vi "Main.vi"(11 "Module Admin":refnum<class "Delacor_lib_QMH_Module Admin.lvclass">) -> ()   [LabVIEW 2020, in "Logger.lvlib"]
doc: "This template is based off of the Queued Message Handler design pattern and the Queued Message Handler project template that ships with LabVIEW.\n\nThe main difference is that the queue is private to this module and communication between modules is performed via Broadcast and Request events.\n\nRequest events are wrapped in public API methods and are handled in the Event Handling Loop (EHL) of this VI. Any module can register for Broadcast events sent by this module. The EHL generates messages based on user interface actions.\n\nThe Message Handling Loop (MHL) processes messages generated by the EHL, or by other messages. The messages are string values, so new messages can be added easily to the Message Cases case structure in the MHL. Each message cluster can also provide an optional value for Message Data, which is a variant that can be converted to whatever message-specific data is required.\n_____\nBased on Delacor QMH Project Template 4.0.0.47.\n_____\nBased on DQMH Project Template 6.0.0.91."
uses:
  Logger.lvlib
  <vilib>/Delacor/Delacor QMH/Libraries/Module Admin_class/Delacor_lib_QMH_Module Admin.lvclass
  Module Data--cluster.ctl
  Stop Argument--cluster.ctl
  <vilib>/Delacor/Delacor QMH/Libraries/Message Queue_class/Delacor_lib_QMH_Message Queue.lvclass/Delacor_lib_QMH_Message Queue.ctl
  <vilib>/Delacor/Delacor QMH/Libraries/Module Admin_class/Delacor_lib_QMH_Module Admin.lvclass/Delacor_lib_QMH_Module Admin.ctl
  Initialize File Argument--cluster.ctl
  Initialize File (Reply Payload)--cluster.ctl
  Log Data Argument--cluster.ctl
  Stop Logging Argument--cluster.ctl
  Settings Editor/Update Application Settings (Reply Payload)--cluster.ctl
  Settings Editor/Settings--cluster.ctl
  Settings Editor/DAQmx Config--cluster.ctl
  Settings Editor/DAQmx Trigger Settings--cluster.ctl
  Settings Editor/DAQmx Timing--cluster.ctl
  Start Logging Argument--cluster.ctl
  <vilib>/Utility/miscctls.llb/LVPointTypeDef.ctl
  <vilib>/Delacor/Delacor QMH/Libraries/Message Queue_class/Delacor_lib_QMH_Enqueue Message (Single).vi
  <vilib>/Delacor/Delacor QMH/Libraries/Module Admin_class/Delacor_lib_QMH_Get External Launch.vi
  <vilib>/Utility/error.llb/Error Cluster From Error Code.vi
  <vilib>/ErrorRing/Error Ring.xnode
  <vilib>/Delacor/Delacor QMH/Libraries/Message Queue_class/Delacor_lib_QMH_Message Queue.lvclass
  Settings Editor/Settings Editor.lvlib
panel:
  out "Settings":T1
  out "error out":errorcluster
  # "This is a headless module. Show its panel to confirm that the Settings are updated correctly and other debugging tasks. Use the Settings Editor to change the settings for this module."
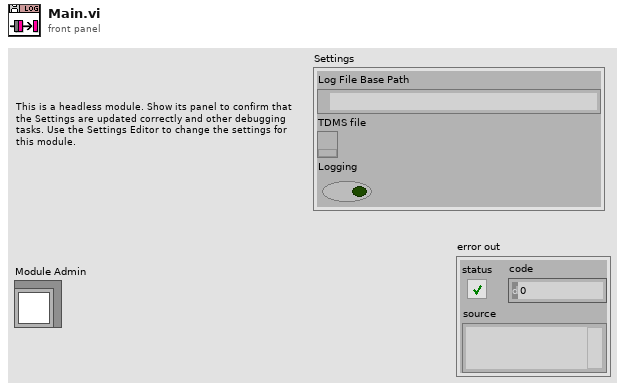
[diagram p1: front panel]
types:
  T1 = typedef "Logger.lvlib/Module Data--cluster.ctl" = cluster{"Log File Base Path":path, "TDMS file":refnum<k34>, "Logging":bool}
  T2 = typedef "Settings Editor.lvlib/Broadcast Events--cluster.ctl" = cluster{"Module Did Init":refnum<user-event>, "Status Updated":refnum<user-event>, "Error Reported":refnum<user-event>, "Module Did Stop":refnum<user-event>, "Update Module Execution Status":refnum<user-event>, "Application Settings Updated":refnum<user-event>}
  T3 = typedef "Logger.lvlib/Request Events--cluster.ctl" = cluster{"Stop Module":refnum<user-event>, "Show Panel":refnum<user-event>, "Hide Panel":refnum<user-event>, "Get Module Execution Status":refnum<user-event>, "Show Diagram":refnum<user-event>, "Stop Logging":refnum<user-event>, "Log Data":refnum<user-event>, "Initialize File":refnum<user-event>, "Start Logging":refnum<user-event>}
  T4 = enum32{"invalid lock state", "Not Locked", "Locked (No Password)", "Password-protected"}
  T5 = typedef "Logger.lvlib/Stop Argument--cluster.ctl" = cluster{"Origin":string, "Exit via Stop Module Req?":bool, "Wait for Module to stop?":bool}
  T6 = typedef "Logger.lvlib/Initialize File Argument--cluster.ctl" = cluster{"Wait Notifier":refnum<notifier>, "wait for reply":bool}
  T7 = typedef "Logger.lvlib/Log Data Argument--cluster.ctl" = cluster{"Waveforms":waveform(dbl)[]}
  T8 = typedef "Logger.lvlib/Stop Logging Argument--cluster.ctl" = cluster{"Boolean":bool}
  T9 = typedef "Settings Editor.lvlib/Update Application Settings (Reply Payload)--cluster.ctl" = cluster{"Settings":T10, "Update Settings_error":errorcluster}
  T10 = typedef "Settings Editor.lvlib/Settings--cluster.ctl" = cluster{"Calibration Array":cluster{"Slope":dbl, "Offset":dbl}[], "Hardware Config Cluster":T11, "Trigger Settings":T12, "Log File Base Path":path, "DAQmx Timing Settings":T13}
  T11 = typedef "Settings Editor.lvlib/DAQmx Config--cluster.ctl" = cluster{"Physical channels":tag, "Channel Name":string, "Unit":i32, "Min Voltage":dbl, "Max Voltage":dbl}[]
  T12 = typedef "Settings Editor.lvlib/DAQmx Trigger Settings--cluster.ctl" = cluster{"Trigger Type":enum32{"No Trigger", "Digital Start", "Digital Pause", "Digital Reference", "Analog Start", "Analog Pause", "Analog Reference", "Time Start"}, "Digital Start":cluster{"Source":tag, "Digital Start Trigger Edge":i32}, "Digital Pause":cluster{"Source":tag, "Digital Pause Trigger Pause When":i32}, "Digital Reference":cluster{"Source":tag, "Digital Start Trigger Edge":i32, "Digital Reference Pretrigger Samples":u32}, "Analog Start":cluster{"Source":string, "Analog Slope":i32, "Analog Start Trigger Hysteresis":dbl, "Analog Start Trigger Level":dbl}, "Analog Pause":cluster{"Source":string, "Analog Start Trigger Level":dbl, "Analog Pause Trigger Pause When":i32}, "Analog Reference":cluster{"Source":string, "Slope":i32, "Pretrigger Samples":u32, "Level":dbl}, "Time Start":cluster{"Select Time\nManually":bool, "When":timestamp}}
  T13 = typedef "Settings Editor.lvlib/DAQmx Timing--cluster.ctl" = cluster{"rate":dbl, "source":tag, "sample mode":i32, "samples per channel":i32}
  T14 = typedef "Logger.lvlib/Start Logging Argument--cluster.ctl" = cluster{"Boolean":bool}
  T15 = typedef "LVPointTypeDef.ctl" = cluster{"Horizontal":i16, "Vertical":i16}
  T16 = enum32{"Invalid", "Standard", "Closed", "Hidden", "Minimized", "Maximized"}
  T17 = typedef "Logger.lvlib/Initialize File (Reply Payload)--cluster.ctl" = cluster{"File Path":path, "Initialize File_error":errorcluster}
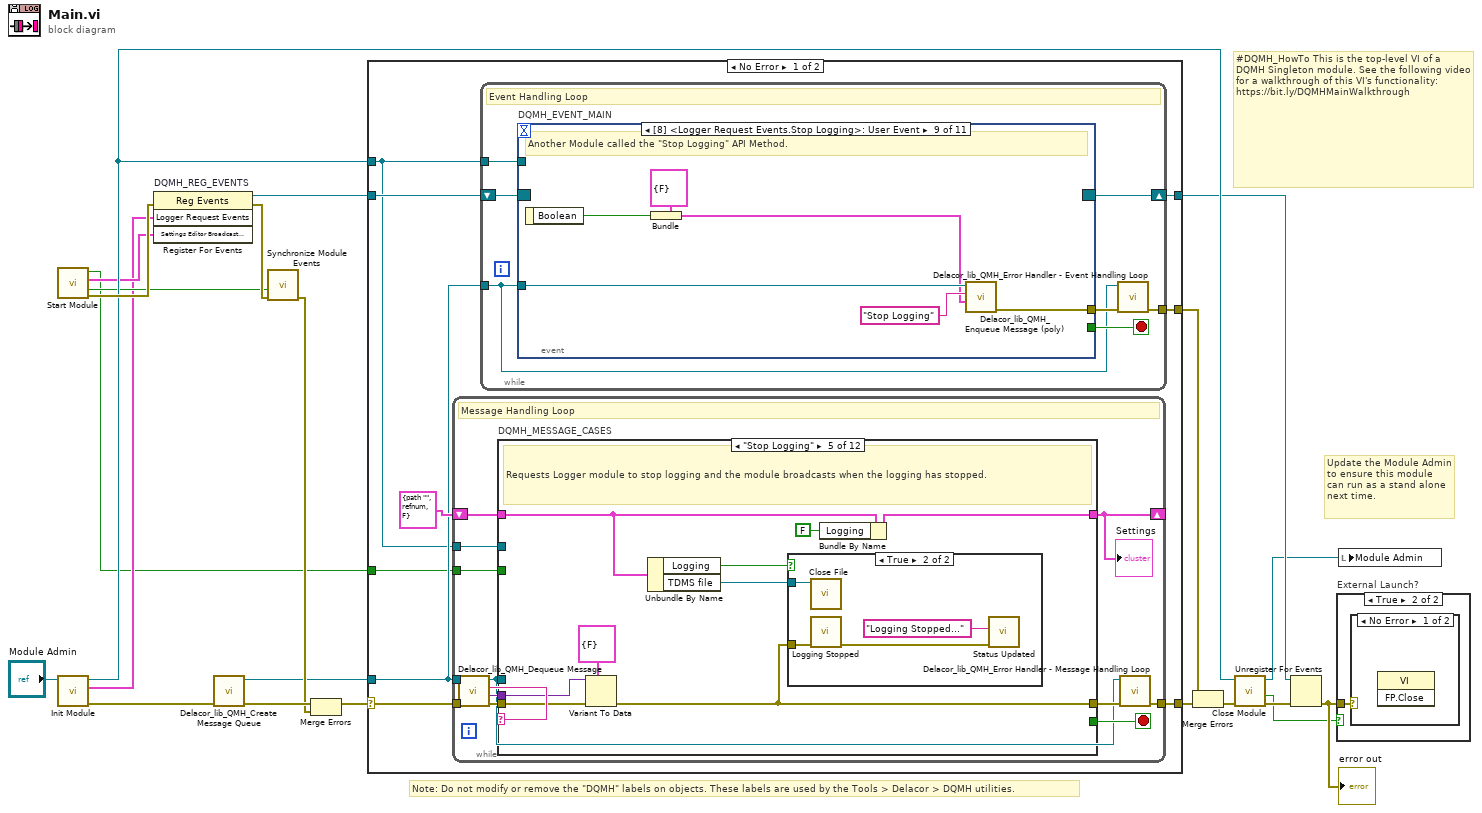
[diagram p0: block diagram]
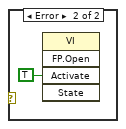
[diagram p3: hidden frame]
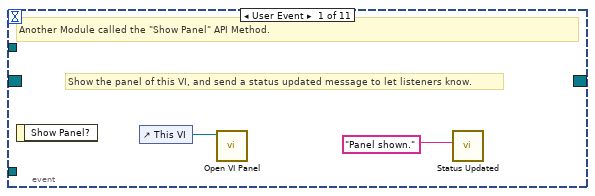
[diagram p4: hidden frame]
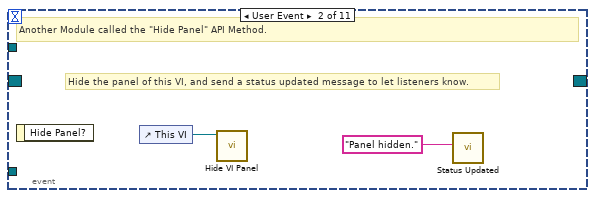
[diagram p5: hidden frame]
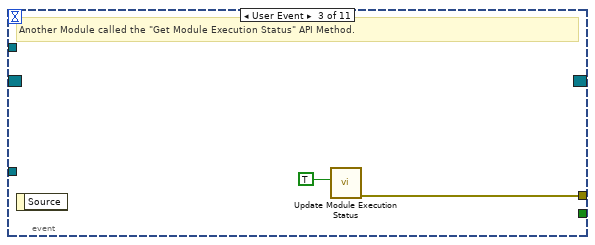
[diagram p6: hidden frame]
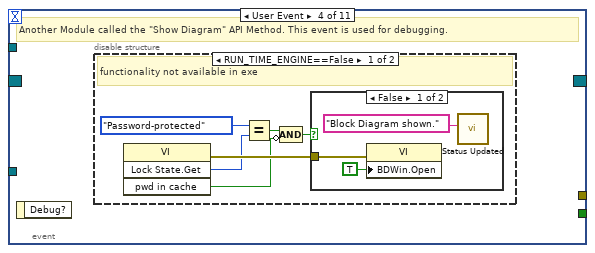
[diagram p7: hidden frame]
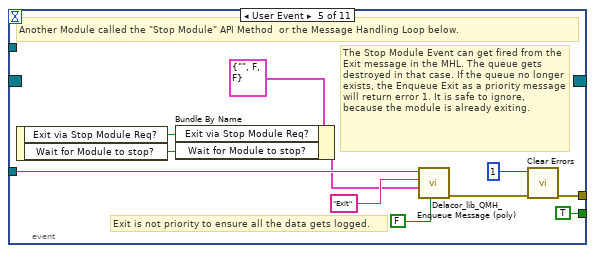
[diagram p10: hidden frame]
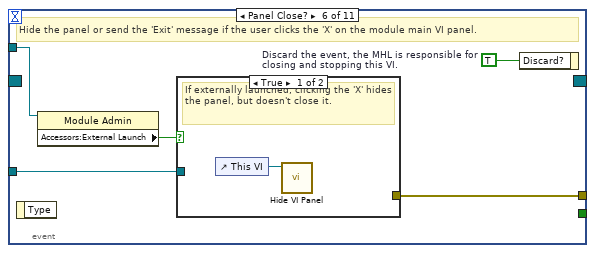
[diagram p11: hidden frame]
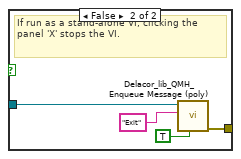
[diagram p12: hidden frame]
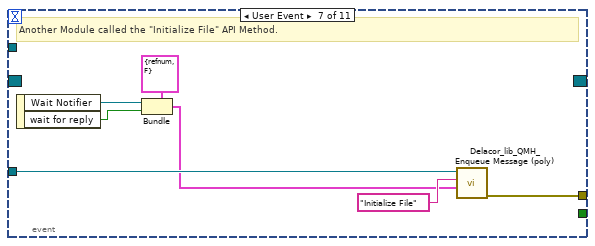
[diagram p13: hidden frame]
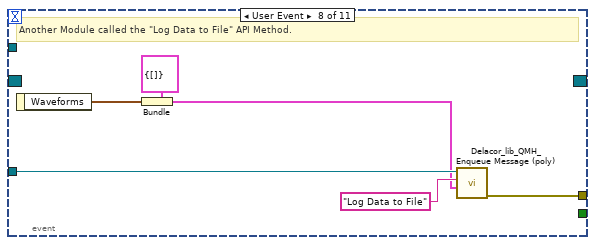
[diagram p14: hidden frame]
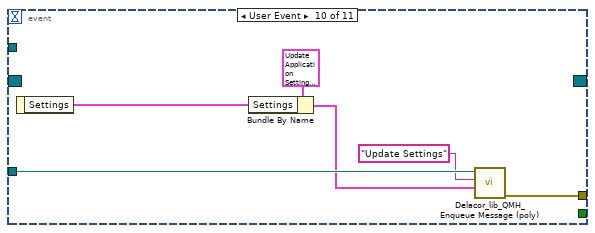
[diagram p15: hidden frame]
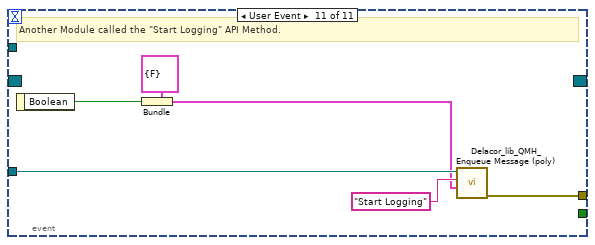
[diagram p16: hidden frame]
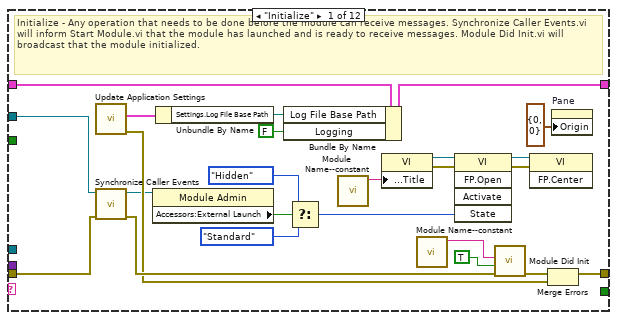
[diagram p17: hidden frame]
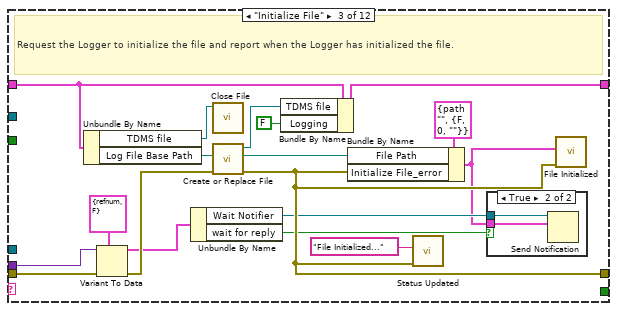
[diagram p19: hidden frame]
diagram:
  # "#DQMH_HowTo This is the top-level VI of a DQMH Singleton module. See the following video for a walkthrough of this VI's functionality: https://bit.ly/DQMHMainWalkthrough"
  # "Note: Do not modify or remove the \"DQMH\" labels on objects. These labels are used by the Tools > Delacor > DQMH utilities."
  # "Update the Module Admin to ensure this module can run as a stand alone next time."
  n1 = call "Start Module.vi"() -> ("error out"=w14:errorcluster, "Wait for Event Sync?"=w4:bool, "Settings Editor Broadcast Events"=w3:T2, "Module Was Already Running?"=w1:bool)  [unwired: 8 in]
  n2 = call "Init Module.vi"("Singleton Module Admin in"="Module Admin") -> ("error out"=w21:errorcluster, "Logger Request Events"=w2:T3, "Singleton Module Admin out"=w11:refnum<class "Delacor_lib_QMH_Module Admin.lvclass">)  [unwired: 8 in]
  n3 = register-events "DQMH_REG_EVENTS"(error in=w14, w2, w3) -> (reference out=w9:refnum<event-registration>, error out=w13:errorcluster)  [unwired: 1 in]
  n4 = call <vilib>:"Delacor_lib_QMH_Create Message Queue.vi"("error in"=w21) -> ("error out"=w16:errorcluster, "Message Queue"=w8:refnum<class "Delacor_lib_QMH_Message Queue.lvclass">)  [unwired: 9 in]
  n5 = call "Synchronize Module Events.vi"("error in (no error)"=w13, "Wait for Event Sync?"=w4) -> ("error out"=w12:errorcluster)  [unwired: 9 in]
  n6 = Merge Errors(w16, w12) -> (w15:errorcluster)
  n7 = case shown="No Error" w15 {
    selector: w15 -> [w29 w267]
    tunnel: [w31 w266] -> w22
    tunnel: [w28 w274] -> w10
    tunnel: w9 -> [w26 w274]
    tunnel: w8 -> [w25 w268]
    tunnel: [w30 _] -> w19
    tunnel: w11 -> [w24 w270]
    tunnel: w1 -> [w23 w269]
    frame No Error {
      n8 = while {
        tunnel: w25 -> [w109]
        shift-right: [w113] -> _
        shift-left: T1 {"Log File Base Path"=path "", "TDMS file"=refnum, "Logging"=FALSE} ("Data Cluster") -> [w114]
        tunnel: w29 -> [w117]
        tunnel: [w115] -> w31
        tunnel: w24 -> [w107]
        tunnel: w23 -> [w106]
        stop <- w112 stop-if-true
        # "Message Handling Loop"
        n9 = call-dynamic "Delacor_lib_QMH_Dequeue Message.vi"("error in"=w117, "Message Queue in"=w109) -> ("error out"=w116:errorcluster, "Message Data"=w110:variant, "Message"=w111:string, "Message Queue out"=w108:refnum<class "Delacor_lib_QMH_Message Queue.lvclass">)  [unwired: 6 in]
        n10 = case "DQMH_MESSAGE_CASES" shown="\"Stop Logging\"" w111 {
          selector: w111 -> [_ _ _ _ _ _ _ _ _ _ _ w253]
          tunnel: w108 -> [_ _ _ _ _ _ _ _ _ w219 w243 _]
          tunnel: w116 -> [w140 w144 w161 w174 w183 w196 w206 w214 w216 w226 w249 w255]
          tunnel: [w137 w144 w162 w170 w182 w189 w204 w213 w216 w222 w246 w256] -> w118
          tunnel: w114 -> [w127 w143 w150 w167 w179 w195 w199 w212 w215 w221 w235 w254]
          tunnel: [w121 w143 w149 w166 w176 w193 w199 w212 w215 w221 w235 w254] -> w113
          tunnel: [_ _ _ _ _ _ _ _ _ _ w242 _] -> w112
          tunnel: w110 -> [_ _ w159 w173 w181 w194 w203 _ _ w220 w241 _]
          tunnel: w107 -> [w128 _ _ _ _ _ _ _ _ w218 w236 _]
          tunnel: w106 -> [_ _ _ _ _ _ _ _ _ _ w233 _]
          frame "Initialize" {
            # "Initialize - Any operation that needs to be done before the module can receive messages. Synchronize Caller Events.vi will inform Start Module.vi that the module has launched and is ready to receive messages. Module Did Init.vi will broadcast that the module initialized."
            n11 = call "Update Application Settings.vi"() -> ("error out"=w136:errorcluster, "Reply Payload"=w122:T9)  [unwired: 9 in, 1 out]
            n12 = call "Synchronize Caller Events.vi"("error in (no error)"=w140, "Singleton Module Admin in"=w128) -> ("error out"=w139:errorcluster, "Singleton Module Admin out"=w124:refnum<class "Delacor_lib_QMH_Module Admin.lvclass">)  [unwired: 8 in]
            n13 = property class="Module Admin"(reference=w124) -> ("Accessors:External Launch"=w132:bool)  [unwired: 1 in, 2 out]
            n14 = Unbundle By Name(w122) -> ("Settings.Log File Base Path"=w120:path)
            n15 = Bundle By Name(cluster=w127, "Log File Base Path"=w120, "Logging"=FALSE) -> (w121:T1)
            n16 = Select(t=T16."Hidden" ("State"), s=w132, f=T16."Standard" ("State")) -> (s? t:f=w129:T16)
            n17 = call "Module Name--constant.vi"() -> ("Module Name"=w135:string)  [unwired: 11 in]
            n18 = property class="VI"("Front Panel.Title"=w135) -> (reference out=w134:refnum<vi>, error out=w142:errorcluster)  [unwired: 2 in]
            n19 = call "Module Name--constant.vi"() -> ("Module Name"=w125:string)  [unwired: 11 in]
            n20 = invoke class="VI" method="FP.Open"(reference=w134, error in=w142, "State"=w129) -> (reference out=w133:refnum<vi>, error out=w141:errorcluster)  [unwired: 2 in, 3 out]
            n21 = call "Module Did Init.vi"("error in (no error)"=w139, "Initialized?"=TRUE, "Origin"=w125) -> ("error out"=w138:errorcluster)  [unwired: 8 in]
            n22 = invoke class="VI" method="FP.Center"(reference=w133, error in=w141) -> ()  [unwired: 1 in, 3 out]
            n23 = Merge Errors(w138, w136) -> (w137:errorcluster)
            n24 = property on="Pane" class="Pane"("Origin"=T15 {"Horizontal"=0, "Vertical"=0}) -> ()  [unwired: 2 in, 2 out]
          }
          frame "---Module Specific---" {
            # "Separator -- The following cases handle messages specific to this Module."
          }
          frame "Initialize File" {
            # "Request the Logger to initialize the file and report when the Logger has initialized the file."
            n25 = Unbundle By Name(w150) -> ("TDMS file"=w145:refnum<k34>, "Log File Base Path"=w152:path)
            n26 = Variant To Data(error in=w161, type=T6 {"Wait Notifier"=refnum, "wait for reply"=FALSE} ("Initialize File Argument"), Variant=w159) -> (data=w157:T6, error out=w160:errorcluster)
            n27 = Unbundle By Name(w157) -> ("Wait Notifier"=w156:refnum<notifier>, "wait for reply"=w155:bool)
            n28 = call "Close File.vi"("Refnum out"=w145) -> ()  [unwired: 10 in, 1 out]
            n29 = call "Create or Replace File.vi"("error in (no error)"=w160, "Log File Base Path"=w152) -> ("error out"=w162:errorcluster, "File Path"=w148:path, "Refnum out"=w151:refnum<k34>)  [unwired: 7 in]
            n30 = Bundle By Name(cluster=w150, "TDMS file"=w151, "Logging"=FALSE) -> (w149:T1)
            n31 = Bundle By Name(cluster=T17 {"File Path"=path "", "Initialize File_error"={"status"=FALSE, "code"=0, "source"=""}} ("Initialize File (Reply Payload)"), "File Path"=w148, "Initialize File_error"=w162) -> (w153:T17)
            n32 = call "Status Updated.vi"("error in (no error)"=w162, "Status"="File Initialized...") -> ()  [unwired: 9 in, 1 out]
            n33 = case shown="True" w155 {
              tunnel: w156 -> [_ w164]
              tunnel: w153 -> [_ w163]
              frame False {
              }
              frame True {
                n34 = Send Notification(notification=w163, notifier=w164) -> ()  [unwired: 1 in, 2 out]
              }
            }
            n35 = call "File Initialized.vi"("error in (no error)"=w162, "Reply Payload"=w153) -> ()  [unwired: 9 in, 1 out]
          }
          frame "Start Logging" {
            # "Requests Logger module to stop logging and the module broadcasts when the logging has stopped."
            n36 = Variant To Data(error in=w174, type=T14 {"Boolean"=FALSE} ("Start Logging Argument"), Variant=w173) -> (data=w171:T14, error out=w170:errorcluster)
            n37 = Unbundle By Name(w171) -> ()  [unwired: 1 out]
            n38 = call "Logging Started.vi"("error in"=w170) -> ("error out"=w169:errorcluster)  [unwired: 10 in]
            n39 = Bundle By Name(cluster=w167, "Logging"=TRUE) -> (w166:T1)
            n40 = call "Status Updated.vi"("error in (no error)"=w169, "Status"="Logging Started...") -> ()  [unwired: 9 in, 1 out]
          }
          frame "Stop Logging" {
            # "Requests Logger module to stop logging and the module broadcasts when the logging has stopped."
            n41 = Variant To Data(error in=w183, type=T8 {"Boolean"=FALSE} ("Stop Logging Argument"), Variant=w181) -> (error out=w182:errorcluster)  [unwired: 1 out]
            n42 = Unbundle By Name(w179) -> ("Logging"=w178:bool, "TDMS file"=w177:refnum<k34>)
            n43 = case shown="True" w178 {
              tunnel: w182 -> [_ w187]
              tunnel: w177 -> [_ w184]
              frame False {
                # "We were not logging, so this is a no-op."
              }
              frame True {
                n44 = call "Close File.vi"("Refnum out"=w184) -> ()  [unwired: 10 in, 1 out]
                n45 = call "Logging Stopped.vi"("error in (no error)"=w187) -> ("error out"=w186:errorcluster)  [unwired: 10 in]
                n46 = call "Status Updated.vi"("error in (no error)"=w186, "Status"="Logging Stopped...") -> ()  [unwired: 9 in, 1 out]
              }
            }
            n47 = Bundle By Name(cluster=w179, "Logging"=FALSE) -> (w176:T1)
          }
          frame "Update Settings" {
            n48 = Variant To Data(error in=w196, type=T9 {"Settings"={"Calibration Array"=[], "Hardware Config Cluster"=[{"Physical channels"="", "Channel Name"="", "Unit"=1, "Min Voltage"=0.0, "Max Voltage"=0.0}], "Trigger Settings"={"Trigger Type"=enum."No Trigger", "Digital Start"={"Source"="", "Digital Start Trigger Edge"=10280}, "Digital Pause"={"Source"="APFI0", "Digital Pause Trigger Pause When"=10192}, "Digital Reference"={"Source"="", "Digital Start Trigger Edge"=10280, "Digital Reference Pretrigger Samples"=0}, "Analog Start"={"Source"="", "Analog Slope"=10093, "Analog Start Trigger Hysteresis"=0.0, "Analog Start Trigger Level"=0.0}, "Analog Pause"={"Source"="", "Analog Start Trigger Level"=0.0, "Analog Pause Trigger Pause When"=10093}, "Analog Reference"={"Source"="", "Slope"=10280, "Pretrigger Samples"=0, "Level"=0.0}, "Time Start"={"Select Time\nManually"=FALSE, "When"=timestamp(0 s since 1904-01-01)}}, "Log File Base Path"=path "", "DAQmx Timing Settings"={"rate"=1000.0, "source"="OnboardClock", "sample mode"=10178, "samples per channel"=1000}}, "Update Settings_error"={"status"=FALSE, "code"=0, "source"=""}} ("Settings Updated Argument"), Variant=w194) -> (data=w192:T9, error out=w189:errorcluster)
            n49 = Unbundle By Name(w192) -> ("Settings.Log File Base Path"=w191:path)
            n50 = Bundle By Name(cluster=w195, "Log File Base Path"=w191) -> (w193:T1)
            n51 = call "Status Updated.vi"("error in (no error)"=w189, "Status"="Settings Updated") -> ()  [unwired: 9 in, 1 out]
          }
          frame "Log Data to File" {
            # "Requests Logger module to log data to file"
            n52 = Variant To Data(error in=w206, type=T7 {"Waveforms"=[]} ("Log Data to File Argument"), Variant=w203) -> (data=w201:T7, error out=w205:errorcluster)
            n53 = Unbundle By Name(w199) -> ("Logging"=w197:bool, "TDMS file"=w198:refnum<k34>)
            n54 = Unbundle By Name(w201) -> ("Waveforms"=w200:waveform(dbl)[])
            n55 = case shown="True" w197 {
              tunnel: w205 -> [w207 w211]
              tunnel: [w207 w210] -> w204
              tunnel: w200 -> [_ w209]
              tunnel: w198 -> [_ w208]
              frame False {
                # "We are not currently logging, so this action is a no-op."
              }
              frame True {
                n56 = call "Log Data to File.vi"("error in (no error)"=w211, "Data to log"=w209, "TDMS File Reference"=w208) -> ("error out"=w210:errorcluster)  [unwired: 8 in]
              }
            }
          }
          frame "---Copy This Frame---" {
            # "Duplicate this frame when creating new messages.  Change this comment in the duplicated frame to describe this message."
            n57 = Merge Errors(w214) -> (w213:errorcluster)
          }
          frame "---Exit and Error Handling---" {
            # "Separator - The following cases handle errors and exit messages."
          }
          frame "Error" {
            # "Error - Check the error message data and respond accordingly. This message is sent by the \"Error Handler\" VIs at the end of each loop in this application."
            n58 = property class="Module Admin"(reference=w218) -> ("Accessors:External Launch"=w217:bool)  [unwired: 1 in, 2 out]
            n59 = Variant To Data(error in=w226, type=errorcluster {"status"=FALSE, "code"=0, "source"=""} ("error constant"), Variant=w220) -> (data=w227:errorcluster, error out=w224:errorcluster)
            n60 = call "Error Reported.vi"("Error"=w227) -> ()  [unwired: 10 in, 1 out]
            n61 = case shown="False" w217 {
              tunnel: [w232 _] -> w223
              tunnel: w219 -> [w230 _]
              tunnel: w227 -> [w231 _]
              frame False {
                # "If the module is running standalone, then pop up an error dialog and call the \"Exit\" message."
                n62 = call <vilib>:"Simple Error Handler.vi"("error in (no error)"=w231) -> ()  [unwired: 4 in, 5 out]
                n63 = call-poly <vilib>:"Delacor_lib_QMH_Enqueue Message (poly).vi"("Priority Message? (F)"=TRUE, "Message"="Exit", "Message Queue in"=w230) -> ("error out"=w232:errorcluster)  [unwired: 7 in, 1 out]
              }
              frame True {
                # "If the module was launched externally, calling the Error Reported broadcast VI is the only action performed by the \"Error\" message. The module's caller can then process the error appropriately."
              }
            }
            n64 = Merge Errors(w224, w223) -> (w222:errorcluster)
            n65 = local write "error out"(w222) -> ()
          }
          frame "Exit" {
            w240 = 91  # 91: not all Exit messages will have an argument
            w242 = TRUE  # Stop the VI
            # "Release the message queue reference"
            # "Exit - Exit the application."
            n66 = Variant To Data(error in=w249, type=T5 {"Origin"="", "Exit via Stop Module Req?"=FALSE, "Wait for Module to stop?"=FALSE} ("Stop Argument"), Variant=w241) -> (data=w238:T5, error out=w245:errorcluster)
            n67 = call <vilib>:"Clear Errors.vi"("error in (no error)"=w245, "specific error code to clear (0: all)"=w240) -> ("error out"=w248:errorcluster)  [unwired: 4 in, 1 out]
            n68 = Unbundle By Name(w235) -> ("TDMS file"=w234:refnum<k34>)
            n69 = control-ref of="This VI"() -> (w237:refnum<vi>)
            n70 = call-dynamic "Delacor_lib_QMH_Release Message Queue.vi"("error in"=w248, "Message Queue"=w243) -> ("error out"=w247:errorcluster)  [unwired: 9 in]
            n71 = call "Handle Exit.vi"("Stop Argument"=w238, "Admin in"=w236, "VI reference"=w237) -> ("error out"=w244:errorcluster)  [unwired: 7 in, 1 out]
            n72 = call "Close File.vi"("Refnum out"=w234) -> ()  [unwired: 10 in, 1 out]
            n73 = case "Settings Editor was\nalready running?" shown="False" w233 {
              frame False {
                n74 = call "Module Name--constant.vi"() -> ("Module Name"=w251:string)  [unwired: 11 in]
                n75 = call "Stop Module.vi"("Wait for Module to Stop? (F)"=TRUE, "Origin"=w251) -> ()  [unwired: 9 in, 1 out]
              }
              frame True {
                # "Another Module is\nin charge of stopping Settings Editor"
              }
            }
            n76 = Merge Errors(w247, w244) -> (w246:errorcluster)
          }
          frame Default {
            # "'Default' case only runs if there is a message that isn't defined in any of the other cases.  Output a programming error."
            n77 = call "Module Name--constant.vi"() -> ("Module Name"=w252:string)  [unwired: 11 in]
            n78 = xnode "Error Ring"("parameter 0"=w253, "parameter 1"=w252) -> ("error out"=w257:errorcluster)
            n79 = Merge Errors(w255, w257) -> (w256:errorcluster)
          }
        }
        "Settings" <- w113
        n80 = call-dynamic "Delacor_lib_QMH_Error Handler - Message Handling Loop.vi"("error in"=w118, "Message Queue in"=w108) -> ("dup error in"=w115:errorcluster)  [unwired: 8 in, 1 out]
      }
      n81 = while {
        tunnel: w25 -> [w32]
        shift-right: [w35] -> w28
        shift-left: w26 -> [w36]
        tunnel: [w37] -> w30
        tunnel: w24 -> [w33]
        stop <- w34 stop-if-true
        # "Event Handling Loop"
        n82 = event "DQMH_EVENT_MAIN" shown="[8] <Logger Request Events.Stop Logging>: User Event" {
          selector: w36 -> [_ _ _ _ _ _ _ _ _ _ _]
          dyn-events: [_ _ _ _ _ _ _ _ _ _ _] -> w35
          timeout: _ -> [_ _ _ _ _ _ _ _ _ _ _]
          tunnel: [_ _ _ _ TRUE ("Discard?") _ _ _ _ _ _] -> w34
          tunnel: w32 -> [_ _ _ _ w60 w67 w80 w86 w92 w98 w105]
          tunnel: [_ _ w44 _ w63 w69 w81 w87 w93 w99 w100] -> w38
          tunnel: w33 -> [_ _ _ _ _ w66 _ _ _ _ _]
          event User Event {
            # "Show the panel of this VI, and send a status updated message to let listeners know."
            # "Another Module called the \"Show Panel\" API Method."
            n83 = event-data() -> ()  [unwired: 1 in, 1 out]
            n84 = control-ref of="This VI"() -> (w40:refnum<vi>)
            n85 = call "Open VI Panel.vi"("VI"=w40) -> ()  [unwired: 10 in, 1 out]
            n86 = call "Status Updated.vi"("Status"="Panel shown." ("format string")) -> ()  [unwired: 10 in, 1 out]
          }
          event User Event {
            # "Hide the panel of this VI, and send a status updated message to let listeners know."
            # "Another Module called the \"Hide Panel\" API Method."
            n87 = event-data() -> ()  [unwired: 1 in, 1 out]
            n88 = control-ref of="This VI"() -> (w42:refnum<vi>)
            n89 = call "Hide VI Panel.vi"("VI"=w42) -> ()  [unwired: 10 in, 1 out]
            n90 = call "Status Updated.vi"("Status"="Panel hidden." ("format string")) -> ()  [unwired: 10 in, 1 out]
          }
          event User Event {
            # "Another Module called the \"Get Module Execution Status\" API Method."
            n91 = event-data() -> ()  [unwired: 1 in, 1 out]
            n92 = call "Update Module Execution Status.vi"("Running?"=TRUE) -> ("error out"=w44:errorcluster)  [unwired: 10 in]
          }
          event User Event {
            # "Another Module called the \"Show Diagram\" API Method. This event is used for debugging."
            n93 = event-data() -> ()  [unwired: 1 in, 1 out]
            n94 = disable-structure shown="RUN_TIME_ENGINE==False" {
              frame condition #0 (active) {
                # "functionality not available in exe"
                n95 = invoke class="VI" method="Lock State.Get"() -> (error out=w50:errorcluster, "Get Lock State"=w49:T4, "pwd in cache"=w46:bool)  [unwired: 4 in, 1 out]
                n96 = Equal?(x=T4."Password-protected", y=w49) -> (x = y?=w47:bool)
                n97 = Compound Arithmetic op=AND(w47, invert w46) -> (w45:bool)
                n98 = case shown="False" w45 {
                  tunnel: w50 -> [w53 _]
                  frame False {
                    n99 = property class="VI"(error in=w53, "BDWin.Open"=TRUE ("Block Diagram Window:Open")) -> ()  [unwired: 1 in, 2 out]
                    n100 = call "Status Updated.vi"("Status"="Block Diagram shown." ("format string")) -> ()  [unwired: 10 in, 1 out]
                  }
                  frame True {
                    # "Password-protected VI, and the password is not in the cache. Do not show the diagram."
                  }
                }
              }
              frame condition #1 {
              }
            }
          }
          event User Event {
            # "Exit is not priority to ensure all the data gets logged."
            # "The Stop Module Event can get fired from the Exit message in the MHL. The queue gets destroyed in that case. If the queue no longer exists, the Enqueue Exit as a priority message will return error 1. It is safe to ignore, because the module is already exiting."
            # "Another Module called the \"Stop Module\" API Method  or the Message Handling Loop below."
            n101 = event-data() -> ("Exit via Stop Module Req?"=w56:bool, "Wait for Module to stop?"=w55:bool)  [unwired: 1 in]
            n102 = Bundle By Name(cluster=T5 {"Origin"="", "Exit via Stop Module Req?"=FALSE, "Wait for Module to stop?"=FALSE} ("Stop Argument"), "Exit via Stop Module Req?"=w56, "Wait for Module to stop?"=w55) -> (w54:T5)
            n103 = call-poly <vilib>:"Delacor_lib_QMH_Enqueue Message (poly).vi"("Priority Message? (F)"=FALSE, "Message Data"=w54, "Message"="Exit", "Message Queue in"=w60) -> ("error out"=w64:errorcluster)  [unwired: 6 in, 1 out]
            n104 = call <vilib>:"Clear Errors.vi"("error in (no error)"=w64, "specific error code to clear (0: all)"=1) -> ("error out"=w63:errorcluster)  [unwired: 4 in, 1 out]
          }
          event Panel Close? {
            w68 = TRUE  # Discard the event, the MHL is responsible for closing and stopping this VI.
            # "Hide the panel or send the 'Exit' message if the user clicks the 'X' on the module main VI panel."
            n105 = event-data() -> ()  [unwired: 1 in, 1 out]
            n106 = property class="Module Admin"(reference=w66) -> ("Accessors:External Launch"=w65:bool)  [unwired: 1 in, 2 out]
            n107 = case shown="True" w65 {
              tunnel: w67 -> [_ w73]
              tunnel: [_ w74] -> w69
              frame True {
                # "If externally launched, clicking the 'X' hides the panel, but doesn't close it."
                n108 = control-ref of="This VI"() -> (w70:refnum<vi>)
                n109 = call "Hide VI Panel.vi"("VI"=w70) -> ()  [unwired: 10 in, 1 out]
              }
              frame False {
                # "If run as a stand-alone VI, clicking the panel 'X' stops the VI."
                n110 = call-poly <vilib>:"Delacor_lib_QMH_Enqueue Message (poly).vi"("Priority Message? (F)"=TRUE, "Message"="Exit", "Message Queue in"=w73) -> ("error out"=w74:errorcluster)  [unwired: 7 in, 1 out]
              }
            }
            n111 = event-data("Discard?"=w68) -> ()  [unwired: 1 in, 1 out]
          }
          event User Event {
            # "Another Module called the \"Initialize File\" API Method."
            n112 = event-data() -> ("Wait Notifier"=w76:refnum<notifier>, "wait for reply"=w75:bool)  [unwired: 1 in]
            n113 = Bundle(cluster=T6 {"Wait Notifier"=refnum, "wait for reply"=FALSE} ("Initialize File Argument"), "Wait Notifier"=w76, "wait for reply"=w75) -> (w77:T6)
            n114 = call-poly <vilib>:"Delacor_lib_QMH_Enqueue Message (poly).vi"("Message Data"=w77, "Message"="Initialize File", "Message Queue in"=w80) -> ("error out"=w81:errorcluster)  [unwired: 7 in, 1 out]
          }
          event User Event {
            # "Another Module called the \"Log Data to File\" API Method."
            n115 = event-data() -> ("Waveforms"=w82:waveform(dbl)[])  [unwired: 1 in]
            n116 = Bundle(cluster=T7 {"Waveforms"=[]} ("Log Data to File Argument"), "Waveforms"=w82) -> (w83:T7)
            n117 = call-poly <vilib>:"Delacor_lib_QMH_Enqueue Message (poly).vi"("Message Data"=w83, "Message"="Log Data to File", "Message Queue in"=w86) -> ("error out"=w87:errorcluster)  [unwired: 7 in, 1 out]
          }
          event User Event {
            # "Another Module called the \"Stop Logging\" API Method."
            n118 = event-data() -> ("Boolean"=w88:bool)  [unwired: 1 in]
            n119 = Bundle(cluster=T8 {"Boolean"=FALSE} ("Stop Logging Argument"), "Boolean"=w88) -> (w89:T8)
            n120 = call-poly <vilib>:"Delacor_lib_QMH_Enqueue Message (poly).vi"("Message Data"=w89, "Message"="Stop Logging", "Message Queue in"=w92) -> ("error out"=w93:errorcluster)  [unwired: 7 in, 1 out]
          }
          event User Event {
            n121 = event-data() -> ("Settings"=w95:T10)  [unwired: 1 in]
            n122 = Bundle By Name(cluster=T9 {"Settings"={"Calibration Array"=[], "Hardware Config Cluster"=[{"Physical channels"="", "Channel Name"="", "Unit"=1, "Min Voltage"=0.0, "Max Voltage"=0.0}], "Trigger Settings"={"Trigger Type"=enum."No Trigger", "Digital Start"={"Source"="", "Digital Start Trigger Edge"=10280}, "Digital Pause"={"Source"="APFI0", "Digital Pause Trigger Pause When"=10192}, "Digital Reference"={"Source"="", "Digital Start Trigger Edge"=10280, "Digital Reference Pretrigger Samples"=0}, "Analog Start"={"Source"="", "Analog Slope"=10093, "Analog Start Trigger Hysteresis"=0.0, "Analog Start Trigger Level"=0.0}, "Analog Pause"={"Source"="", "Analog Start Trigger Level"=0.0, "Analog Pause Trigger Pause When"=10093}, "Analog Reference"={"Source"="", "Slope"=10280, "Pretrigger Samples"=0, "Level"=0.0}, "Time Start"={"Select Time\nManually"=FALSE, "When"=timestamp(0 s since 1904-01-01)}}, "Log File Base Path"=path "", "DAQmx Timing Settings"={"rate"=1000.0, "source"="OnboardClock", "sample mode"=10178, "samples per channel"=1000}}, "Update Settings_error"={"status"=FALSE, "code"=0, "source"=""}} ("Settings Updated Argument"), "Settings"=w95) -> (w94:T9)
            n123 = call-poly <vilib>:"Delacor_lib_QMH_Enqueue Message (poly).vi"("Message Data"=w94, "Message"="Update Settings", "Message Queue in"=w98) -> ("error out"=w99:errorcluster)  [unwired: 7 in, 1 out]
          }
          event User Event {
            # "Another Module called the \"Start Logging\" API Method."
            n124 = event-data() -> ("Boolean"=w101:bool)  [unwired: 1 in]
            n125 = Bundle(cluster=T14 {"Boolean"=FALSE} ("Start Logging Argument"), "Boolean"=w101) -> (w102:T14)
            n126 = call-poly <vilib>:"Delacor_lib_QMH_Enqueue Message (poly).vi"("Message Data"=w102, "Message"="Start Logging", "Message Queue in"=w105) -> ("error out"=w100:errorcluster)  [unwired: 7 in, 1 out]
          }
        }
        n127 = call-dynamic "Delacor_lib_QMH_Error Handler - Event Handling Loop.vi"("error in"=w38, "Message Queue in"=w32) -> ("dup error in"=w37:errorcluster)  [unwired: 8 in, 1 out]
      }
    }
    frame Error {
      # "Synchronize Caller Events.vi will inform Start Module.vi that the module has launched and will let the code calling Start Module.vi register for broadcasts and would permit the caller receive the broadcast that an error occurred at launch time."
      n128 = call "Synchronize Caller Events.vi"("Singleton Module Admin in"=w270) -> ("error out"=w275:errorcluster)  [unwired: 9 in, 1 out]
      n129 = call-dynamic "Delacor_lib_QMH_Release Message Queue.vi"("error in"=w267, "Message Queue"=w268) -> ("error out"=w266:errorcluster)  [unwired: 9 in]
      n130 = call "Module Name--constant.vi"() -> ("Module Name"=w273:string)  [unwired: 11 in]
      n131 = case "Settings Editor was\nalready running?" shown="False" w269 {
        frame False {
          n132 = call "Module Name--constant.vi"() -> ("Module Name"=w278:string)  [unwired: 11 in]
          n133 = call "Stop Module.vi"("Wait for Module to Stop? (F)"=TRUE, "Origin"=w278) -> ()  [unwired: 9 in, 1 out]
        }
        frame True {
          # "Another Module is\nin charge of stopping Settings Editor"
        }
      }
      n134 = Format Into String(format string="An error occurred during initialization. %s is no longer running.", w273) -> (resulting string=w271:string)  [unwired: 2 in, 1 out]
      n135 = Merge Errors(w267, w275) -> (w276:errorcluster)
      n136 = call "Error Reported.vi"("Additional Information"=w271, "Error"=w276) -> ()  [unwired: 9 in, 1 out]
    }
  }
  n137 = Merge Errors(w19, w22) -> (w18:errorcluster)
  n138 = call "Close Module.vi"("error in (no error)"=w18, "Module Admin in"=w11) -> ("error out"=w20:errorcluster, "External Launch"=w5:bool, "Module Admin out"=w6:refnum<class "Delacor_lib_QMH_Module Admin.lvclass">)  [unwired: 7 in]
  n139 = Unregister For Events(event registration refnum=w10, error in=w20) -> (error out=w17:errorcluster)
  "error out" <- w17
  n140 = case "External Launch?" shown="True" w5 {
    tunnel: w17 -> [_ w279]
    frame False {
    }
    frame True {
      n141 = case shown="No Error" w279 {
        frame No Error {
          n142 = invoke class="VI" method="FP.Close"() -> ()  [unwired: 3 in, 3 out]
        }
        frame Error {
          n143 = invoke class="VI" method="FP.Open"("Activate"=TRUE ("Activate?")) -> ()  [unwired: 4 in, 5 out]
        }
      }
    }
  }
  n144 = local write "Module Admin"(w6) -> ()
